vi "AP2_photoelectron_image_aquisition.vi"() -> ()   [LabVIEW 2023]
panel:
  in  "Tab Control":enum32{"PES Acquisition Controls and Montoring"}(tab)
  in  "Stop Control":bool
  in  "Save Image Button":bool
  in  "Discard Image Button":bool
  out "B Counts/5F":dbl
  out "Avg Counts/F":dbl
  out "A Counts":u32
  out "B Counts":u32
  out "Total Counts":u32
  out "FPS":dbl
  in  "Threshold range":cluster{"Lower value":sgl, "Upper value":sgl}={"Lower value"=6.0, "Upper value"=1024.0}
  in  "Region of interest":i32[](array[numeric])
  in  "Number of buffers":u32
  in  "Frame timeout (ms)":u32=1000
  in  "calc R pixel":bool
  in  "Center X":dbl=548.0
  in  "Center Y":dbl=555.0
  in  "update img":bool
  out "A Counts/5F":dbl
  out "Accumulated Image":i16[][](graph)
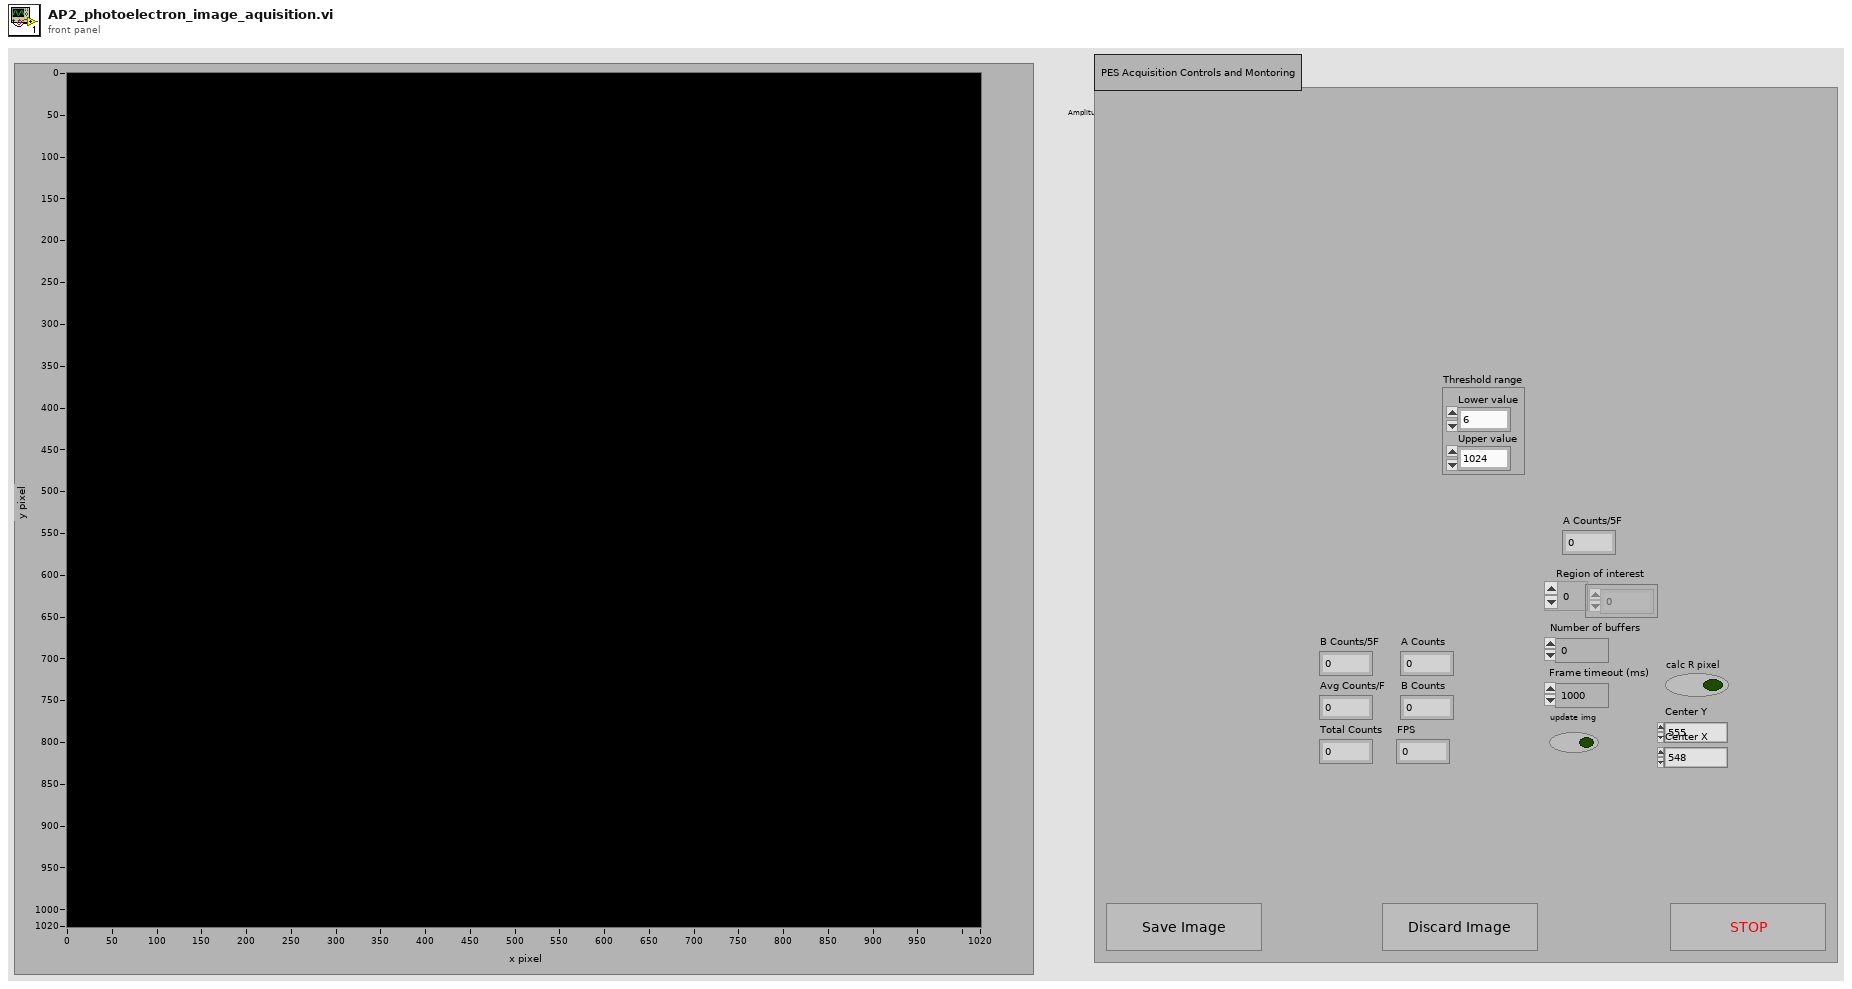
[diagram p1: front panel]
types:
  T1 = cluster{"Region of interest":i32[], "Number of buffers":u32, "Frame timeout (ms)":u32}
  T2 = cluster{"queue out":refnum<queue>, "error out":errorcluster}
  T3 = cluster{"i01 data":sgl[][], "i02 data":sgl[][], "Count Buffer Size Out":i32, "Empty Image":i16[][], "Accumulated Image":i16[][], "Corrected Image 1":i16[][], "Corrected Image 2":i16[][], "Total counts":i32, "t_1":i32, "t_2":i32, "t_3":i32, "t_4":i32, "t_5":i32, "t_6":i32, "t_7":i32, "t_8":i32, "t_9":i32, "t_10":i32, "c_1":i32, "c_2":i32, "Region of interest":i32[]}
  T4 = cluster{"Total Counts":u32, "Avg Counts/F":dbl, "B Counts":u32, "A Counts":u32, "A Counts/5F":dbl, "B Counts/5F":dbl}
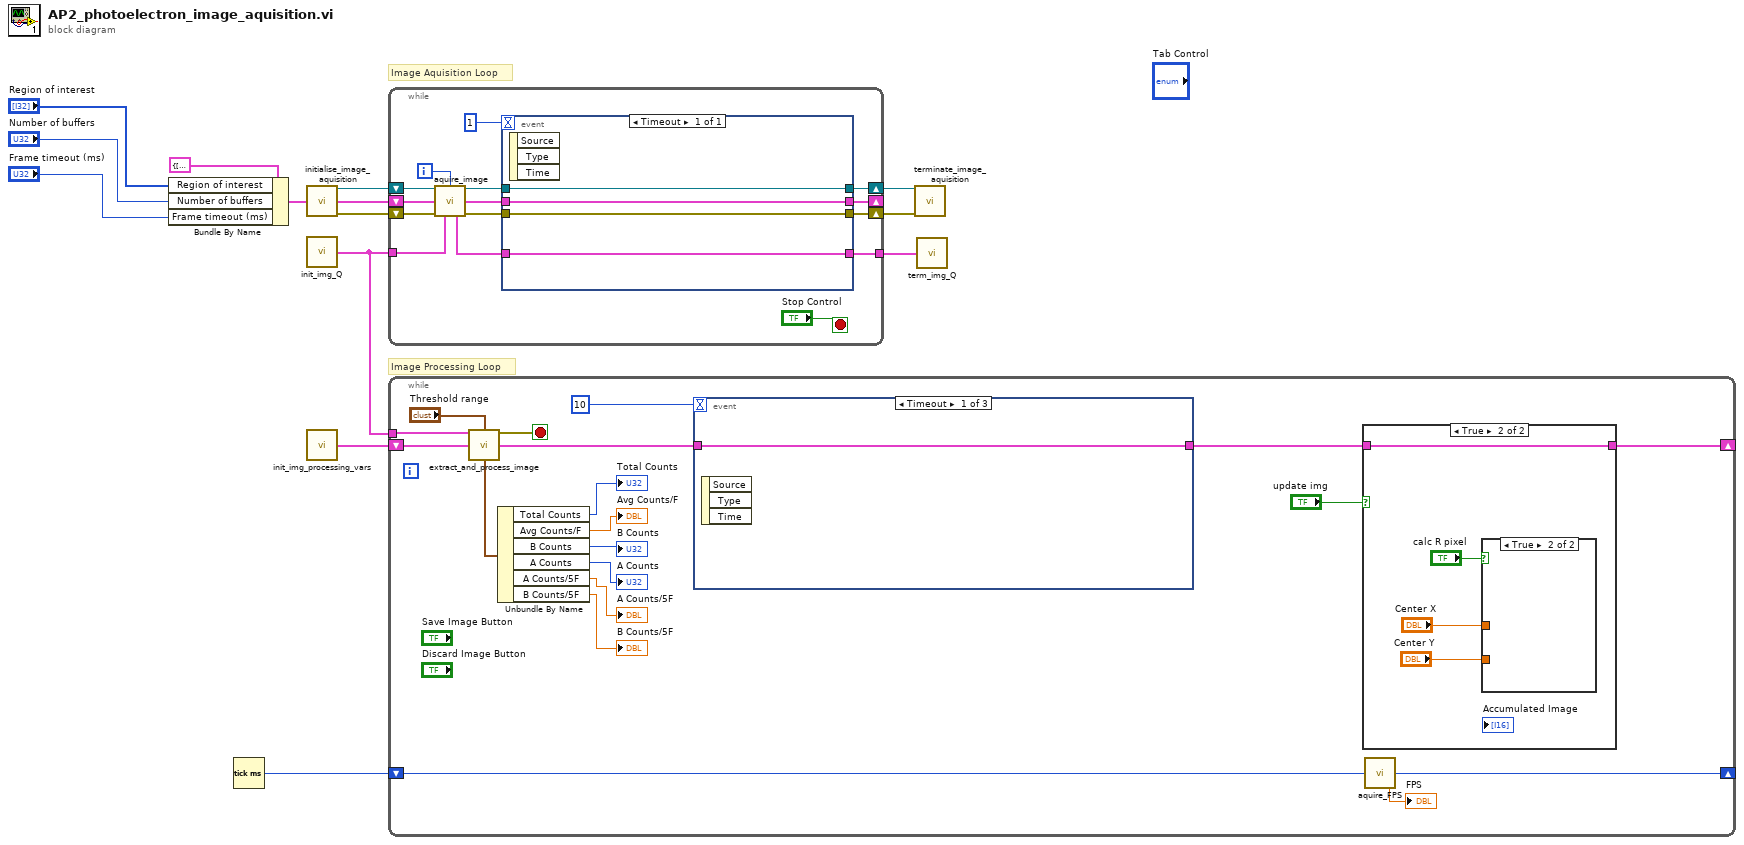
[diagram p0: block diagram]
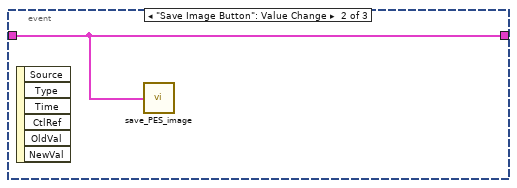
[diagram p2: hidden frame]
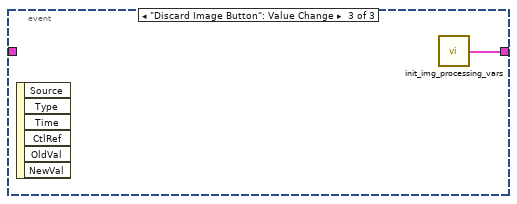
[diagram p3: hidden frame]
diagram:
  # "Image Processing Loop"
  # "Image Aquisition Loop"
  n1 = Bundle By Name(cluster=T1 {"Region of interest"=[], "Number of buffers"=0, "Frame timeout (ms)"=1000}, "Region of interest"="Region of interest", "Number of buffers"="Number of buffers", "Frame timeout (ms)"="Frame timeout (ms)") -> (w8:T1)
  n2 = Tick Count (ms)() -> (millisecond timer value=w2:u32)
  n3 = call "initialise_image_aquisition.vi"("Imaging Variables In"=w8) -> ("IMAQ Session Out"=w14:refnum<k11>, "Imaging Variables Out"=w7:T1, "error out"=w13:errorcluster)  [unwired: 11 in, 1 out]
  n4 = call "init_img_Q.vi"() -> ("Image Q Out"=w5:T2)  [unwired: 15 in]
  n5 = call "init_img_processing_vars.vi"() -> ("Image Processing Data"=w1:T3)  [unwired: 15 in]
  n6 = while {
    shift-right: [w28] -> w4
    shift-left: w14 -> [w25]
    shift-right: [w26] -> w3
    shift-left: w13 -> [w24]
    tunnel: w5 -> [w17]
    tunnel: [w16] -> w6
    shift-right: [w27] -> _
    shift-left: w7 -> [w20]
    i -> [w23]
    stop <- "Stop Control" stop-if-true
    n7 = call "aquire_image.vi"("IMAQ Session In"=w25, "Buffer to extract"=w23, "Imaging Variables In"=w20, "error in (no error)"=w24, "Img Q Data In"=w17) -> ("IMAQ Session Out"=w22:refnum<k11>, "Imaging Variables Out"=w19:T1, "Img Q Data Out"=w18:T2, "error out"=w21:errorcluster)  [unwired: 7 in]
    n8 = event shown="[0] Timeout" {
      selector: _ -> [_]
      dyn-events: _ -> [_]
      timeout: 1 -> [_]
      tunnel: w22 -> [w33]
      tunnel: w21 -> [w32]
      tunnel: [w33] -> w28
      tunnel: [w32] -> w26
      tunnel: w19 -> [w31]
      tunnel: [w31] -> w27
      tunnel: w18 -> [w30]
      tunnel: [w30] -> w16
      event Timeout {
        n9 = event-data() -> ()  [unwired: 1 in, 3 out]
      }
    }
  }
  n10 = while {
    tunnel: w5 -> [w48]
    shift-right: [w50] -> _
    shift-left: w2 -> [w51]
    shift-right: [w45] -> _
    shift-left: w1 -> [w46]
    stop <- w47 stop-if-true
    n11 = call "extract_and_process_image.vi"("Image Q In"=w48, "Threshold range"="Threshold range", "Processed Image Data In"=w46) -> ("error out"=w47:errorcluster, "Processed Image Data Out"=w43:T3, "Count data"=w40:T4)  [unwired: 10 in]
    n12 = Unbundle By Name(w40) -> ("Total Counts"=→"Total Counts":u32, "Avg Counts/F"=→"Avg Counts/F":dbl, "B Counts"=→"B Counts":u32, "A Counts"=→"A Counts":u32, "A Counts/5F"=→"A Counts/5F":dbl, "B Counts/5F"=→"B Counts/5F":dbl)
    n13 = event shown="[0] Timeout" {
      selector: _ -> [_ _ _]
      dyn-events: _ -> [_ _ _]
      timeout: 10 -> [_ _ _]
      tunnel: w43 -> [w53 w54 _]
      tunnel: [w53 w54 w55] -> w41
      event Timeout {
        n14 = event-data() -> ()  [unwired: 1 in, 3 out]
      }
      event "Save Image Button": Value Change {
        n15 = event-data() -> ()  [unwired: 1 in, 6 out]
        n16 = call "save_PES_image.vi"("Processed Image Data In"=w54) -> ()  [unwired: 15 in]
      }
      event "Discard Image Button": Value Change {
        n17 = event-data() -> ()  [unwired: 1 in, 6 out]
        n18 = call "init_img_processing_vars.vi"() -> ("Image Processing Data"=w55:T3)  [unwired: 15 in]
      }
    }
    n19 = case shown="True" "update img" {
      tunnel: w41 -> [w56 w57]
      tunnel: [w56 w57] -> w45
      frame False {
      }
      frame True {
        n20 = case shown="True" "calc R pixel" {
          tunnel: "Center X" -> [_ _]
          tunnel: "Center Y" -> [_ _]
          frame False {
          }
          frame True {
          }
        }
      }
    }
    n21 = call "aquire_FPS.vi"("Time Value In /ms"=w51) -> ("Time Value Out /ms"=w50:u32, "FPS"=→"FPS":dbl)  [unwired: 12 in, 1 out]
  }
  n22 = call "terminate_image_aquisition.vi"("IMAQ Session In"=w4, "error in (no error)"=w3) -> ()  [unwired: 13 in, 1 out]
  n23 = call "term_img_Q.vi"("Image Q Out"=w6) -> ()  [unwired: 14 in, 1 out]
